vi "Test Assert Array Count.vi"(8 "error in (no error)":errorcluster) -> (0 "error out":errorcluster)   [LabVIEW 2013]
uses:
  classes/Assert/Assert.lvclass
  classes/Test/Test.lvclass
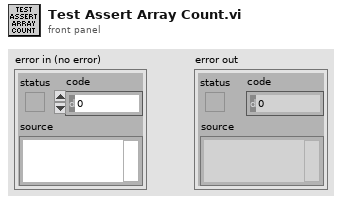
[diagram p1: front panel]
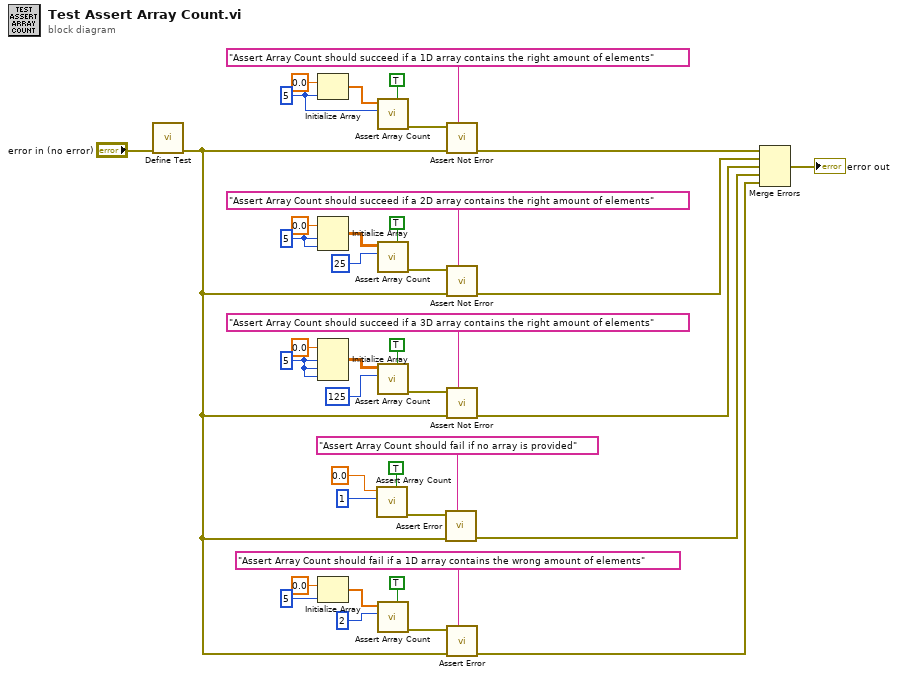
[diagram p0: block diagram]
diagram:
  w17 = 5 ("dimension size")
  w26 = 5 ("dimension size")
  w33 = 5 ("dimension size")
  n1 = call "Define Test.vi"("error in (no error)"="error in (no error)") -> ("error out"=w3:errorcluster)  [unwired: 9 in, 1 out]
  n2 = Initialize Array(0.0 ("element"), w33) -> (w34:dbl[])
  n3 = Initialize Array(0.0 ("element"), w26, w26) -> (w30:dbl[][])
  n4 = Initialize Array(0.0 ("element"), w17, w17, w17) -> (w19:dbl[][][])
  n5 = Initialize Array(0.0 ("element"), 5 ("dimension size")) -> (w7:dbl[])
  n6 = call "Assert Array Count.vi"("Assert Only? (F)"=TRUE, "Count"=1, "Array"=0.0 ("element")) -> ("error out"=w13:errorcluster)  [unwired: 7 in, 1 out]
  n7 = call "Assert Array Count.vi"("Assert Only? (F)"=TRUE, "Count"=w33, "Array"=w34) -> ("error out"=w40:errorcluster)  [unwired: 7 in, 1 out]
  n8 = call "Assert Array Count.vi"("Assert Only? (F)"=TRUE, "Count"=25, "Array"=w30) -> ("error out"=w27:errorcluster)  [unwired: 7 in, 1 out]
  n9 = call "Assert Array Count.vi"("Assert Only? (F)"=TRUE, "Count"=125, "Array"=w19) -> ("error out"=w22:errorcluster)  [unwired: 7 in, 1 out]
  n10 = call "Assert Array Count.vi"("Assert Only? (F)"=TRUE, "Count"=2, "Array"=w7) -> ("error out"=w4:errorcluster)  [unwired: 7 in, 1 out]
  n11 = call "Assert Error.vi"("Label"="Assert Array Count should fail if no array is provided", "error in (no error)"=w3, "Error?"=w13) -> ("error out"=w10:errorcluster)  [unwired: 7 in, 1 out]
  n12 = call "Assert Not Error.vi"("Label"="Assert Array Count should succeed if a 1D array contains the right amount of elements", "error in (no error)"=w3, "Not Error?"=w40) -> ("error out"=w36:errorcluster)  [unwired: 7 in, 1 out]
  n13 = call "Assert Not Error.vi"("Label"="Assert Array Count should succeed if a 2D array contains the right amount of elements", "error in (no error)"=w3, "Not Error?"=w27) -> ("error out"=w24:errorcluster)  [unwired: 7 in, 1 out]
  n14 = call "Assert Not Error.vi"("Label"="Assert Array Count should succeed if a 3D array contains the right amount of elements", "error in (no error)"=w3, "Not Error?"=w22) -> ("error out"=w16:errorcluster)  [unwired: 7 in, 1 out]
  n15 = call "Assert Error.vi"("Label"="Assert Array Count should fail if a 1D array contains the wrong amount of elements", "error in (no error)"=w3, "Error?"=w4) -> ("error out"=w2:errorcluster)  [unwired: 7 in, 1 out]
  n16 = Merge Errors(w36, w24, w16, w10, w2) -> (→"error out":errorcluster)
